vi "Read Synchronization Stuff.vi"(8 "error in (no error)":errorcluster, 11 "IP Connection in":refnum<class "IP Connection.lvclass">) -> (0 "error out":errorcluster, 2 "Synchronization Stuff":T1, 3 "IP Connection out":refnum<class "IP Connection.lvclass">)   [LabVIEW 2011, in "Tinkerforge.lvlib" / "IP Connection.lvclass"]
uses:
  IP Connection.lvclass
  Type Definitions/Sync Stuff.ctl
  Type Definitions/Message.ctl
  Type Definitions/Request Identifier.ctl
  Type Definitions/Answer.ctl
  Type Definitions/Request Type.ctl
  Type Definitions/Enumerate CB.ctl
  Device/Device.lvclass
  IP Connection.lvclass/IP Connection.ctl
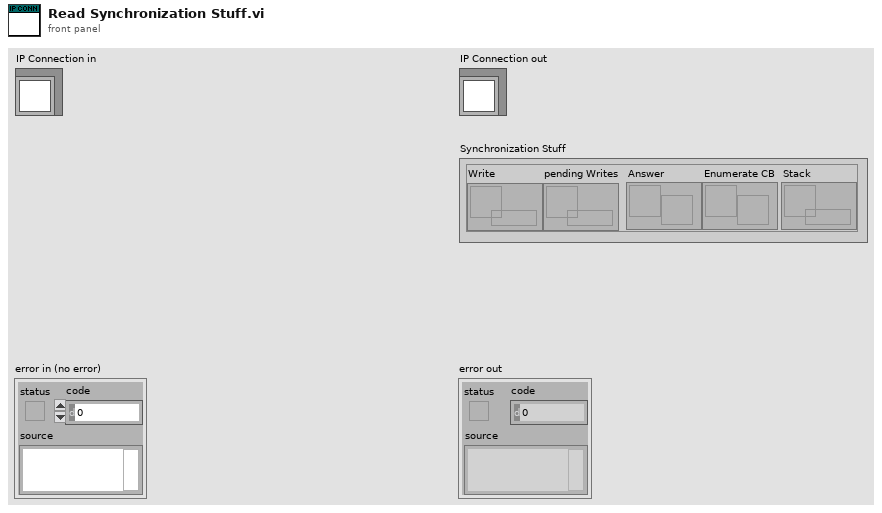
[diagram p1: front panel]
types:
  T1 = typedef "Tinkerforge.lvlib/IP Connection.lvclass/Sync Stuff.ctl" = cluster{"Write":refnum<queue>, "pending Writes":refnum<queue>, "Answer":refnum<user-event>, "Enumerate CB":refnum<user-event>, "Stack":refnum<queue>}
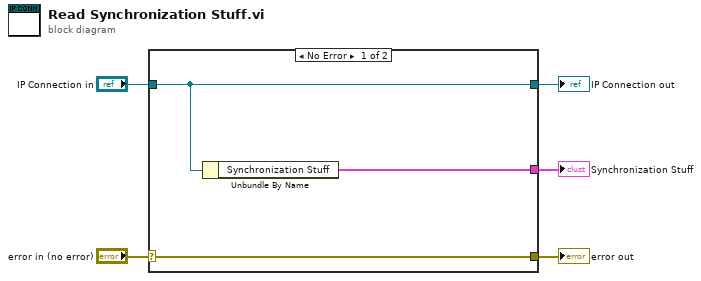
[diagram p0: block diagram]
diagram:
  n1 = case shown="No Error" "error in (no error)" {
    selector: "error in (no error)" -> [w8 w9]
    tunnel: [w8 w9] -> w4
    tunnel: [w7 w10] -> w2
    tunnel: "IP Connection in" -> [w7 w10]
    tunnel: [w6 _] -> w1
    frame No Error {
      n2 = Unbundle By Name(w7) -> ("Synchronization Stuff"=w6:T1)
    }
    frame Error {
    }
  }
  "error out" <- w4
  "IP Connection out" <- w2
  "Synchronization Stuff" <- w1
